vi "gnuplotVectors.vi"(0 "XYUVArray":dbl[][](array[numeric])=[[-138.0, 28.0, -5.0, -3.0], [-92.0, 28.0, -10.0, -5.5], [-46.0, 28.0, -5.0, -10.5], [0.0, 28.0, -9.0, 3.5], [46.0, 28.0, -22.0, 1.0], [92.0, 28.0, -24.5, -9.0], [138.0, 28.0, -16.0, -23.0], [-138.0, 60.0, -6.0, -2.0], [-92.0, 60.0, -7.0, -12.0], [-46.0, 60.0, -6.0, -11.0], [0.0, 60.0, -9.0, 3.0], [46.0, 60.0, -5.5, 6.0], [92.0, 60.0, -10.0, -7.5], [138.0, 60.0, -17.0, -22.0], [-138.0, 92.0, 0.5, 2.0], [-92.0, 92.0, -1.5, -15.0], [-46.0, 92.0, -1.5, -10.5], [0.0, 92.0, 1.0, -1.5], [46.0, 92.0, 1.0, 3.0], [92.0, 92.0, -2.5, -7.5], [138.0, 92.0, -5.0, -17.0], [-138.0, 124.0, 18.5, 15.0], [-92.0, 124.0, 10.5, -2.5], [-46.0, 124.0, 6.5, -2.0], [0.0, 124.0, 7.5, 5.0], [46.0, 124.0, 9.5, 12.5], [92.0, 124.0, 14.0, 8.5], [138.0, 124.0, 6.5, -4.0], [-138.0, 156.0, 13.5, 14.5], [-92.0, 156.0, 19.5, 4.0], [-46.0, 156.0, 12.5, -1.0], [0.0, 156.0, 10.5, 3.5], [46.0, 156.0, 14.0, 11.0], [92.0, 156.0, 17.5, 10.5], [138.0, 156.0, 12.0, -4.5], [-138.0, 188.0, 9.0, 16.5], [-92.0, 188.0, 10.0, 8.0], [-46.0, 188.0, 14.0, 4.0], [0.0, 188.0, 15.5, 8.0], [46.0, 188.0, 14.5, 11.0], [92.0, 188.0, 21.5, 11.0], [138.0, 188.0, 19.0, 0.5], [-138.0, 214.0, 12.5, 11.5], [-92.0, 214.0, 17.5, 6.0], [-46.0, 214.0, 17.0, 9.5], [0.0, 214.0, 14.5, 10.5], [46.0, 214.0, 19.0, 10.5], [92.0, 214.0, 20.0, 7.0], [138.0, 214.0, 16.5, 7.0]] caption="X                    Y                      U                  V", 1 "Job Directory":path) -> (2 "Saved Automatically?":bool, 3 "gnuplotScript":string, 4 "Plot data file":path)   [LabVIEW 2013]
uses:
  Results_plotter_Global.vi
panel:
  in  "OpenLogfile?":bool
  in  "Show Script Editor?":bool
  in  "Tab Control":enum32{"Titles", "OtherStuff ", "TerminalTest"}(tab)=enum."OtherStuff "
  in  "Page Title Pre Block":string
  in  "Page Title Post Block":string
  in  "Values to include in Page Title":i32[](listbox)
  out "Final Title":string
  in  "Filename Max length":i32=255
  out "File Path Control":path
  out "AuditTrail":string[](array[string])
  # "Overall Page Title"
  # "Shows the numbered line colours and point styles available- well it would, if it didn't disappear every time I update from the repository..!"
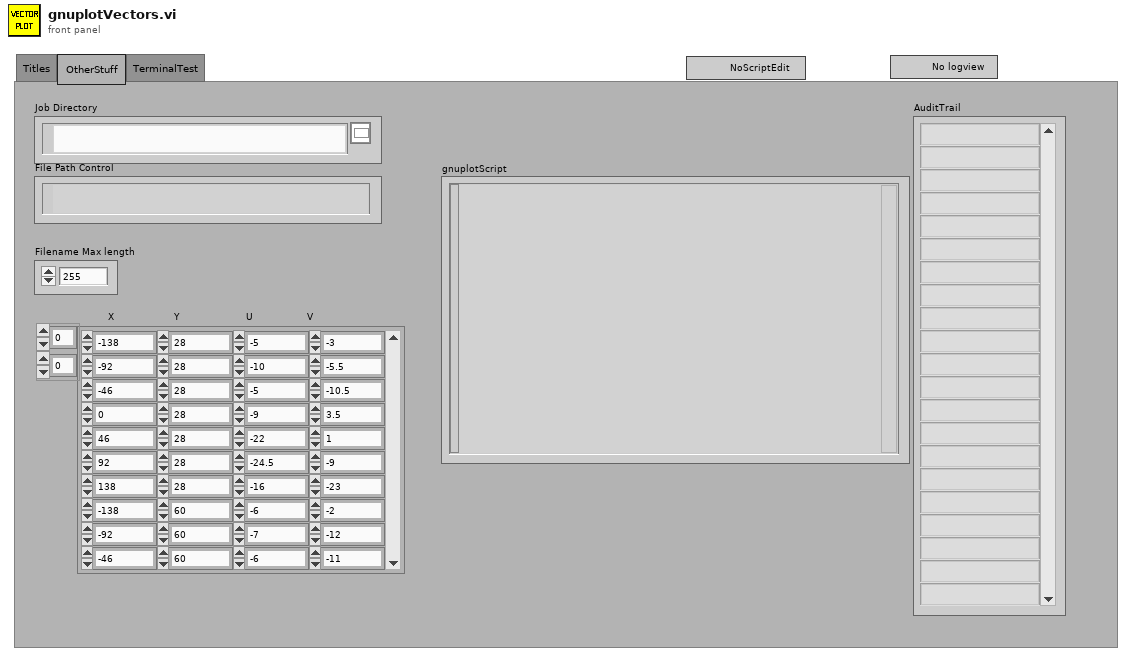
[diagram p1: front panel]
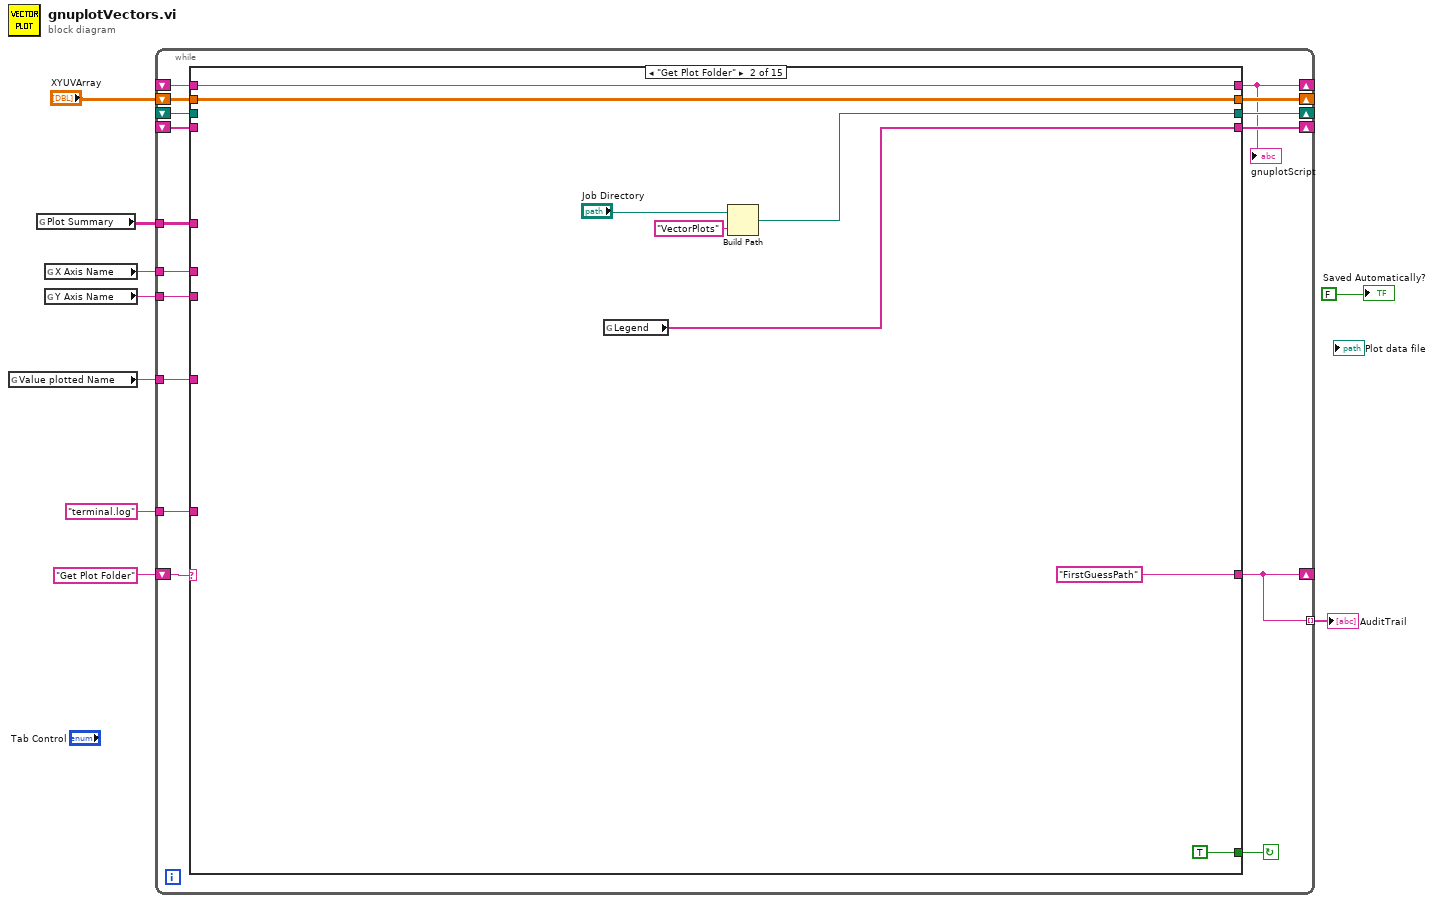
[diagram p0: block diagram]
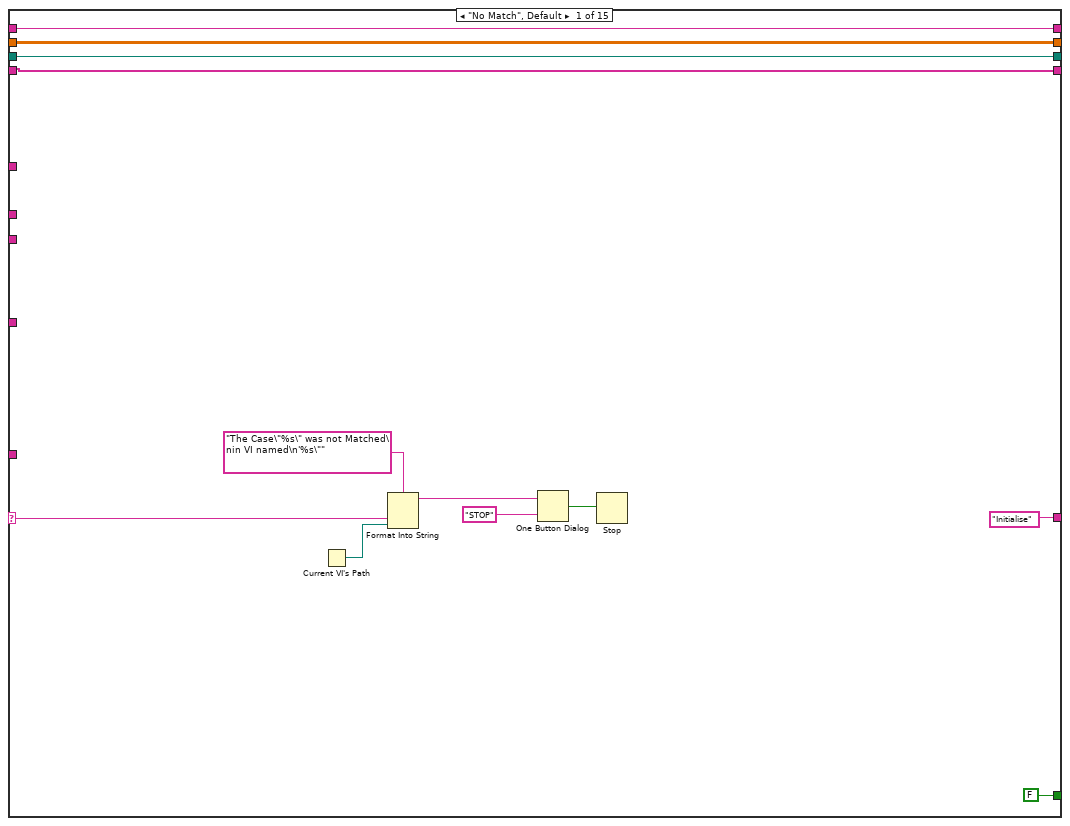
[diagram p2: hidden frame]
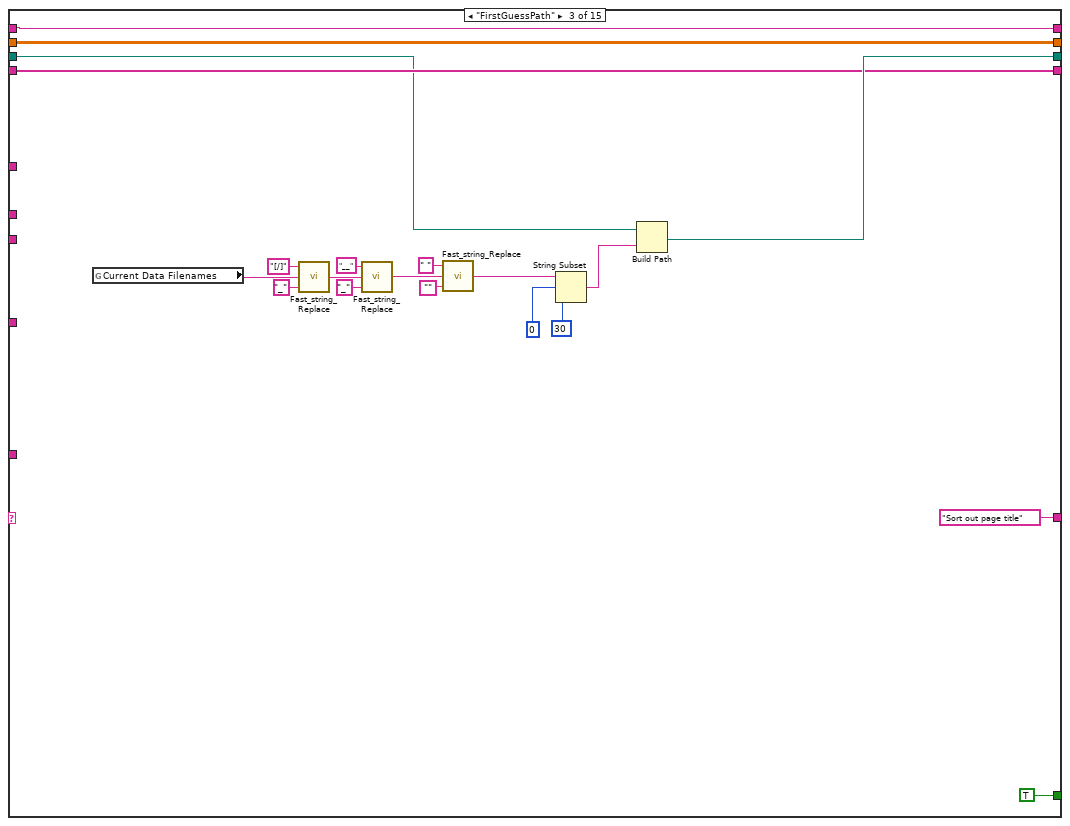
[diagram p3: hidden frame]
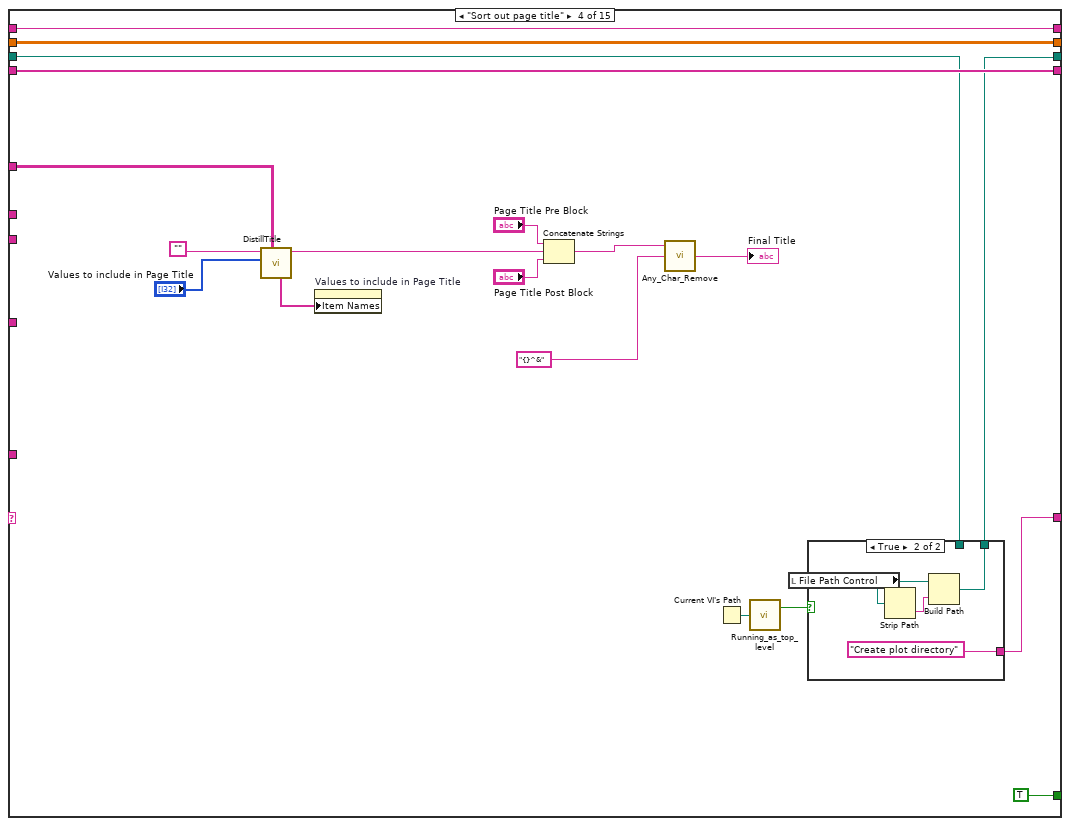
[diagram p4: hidden frame]
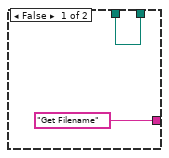
[diagram p5: hidden frame]
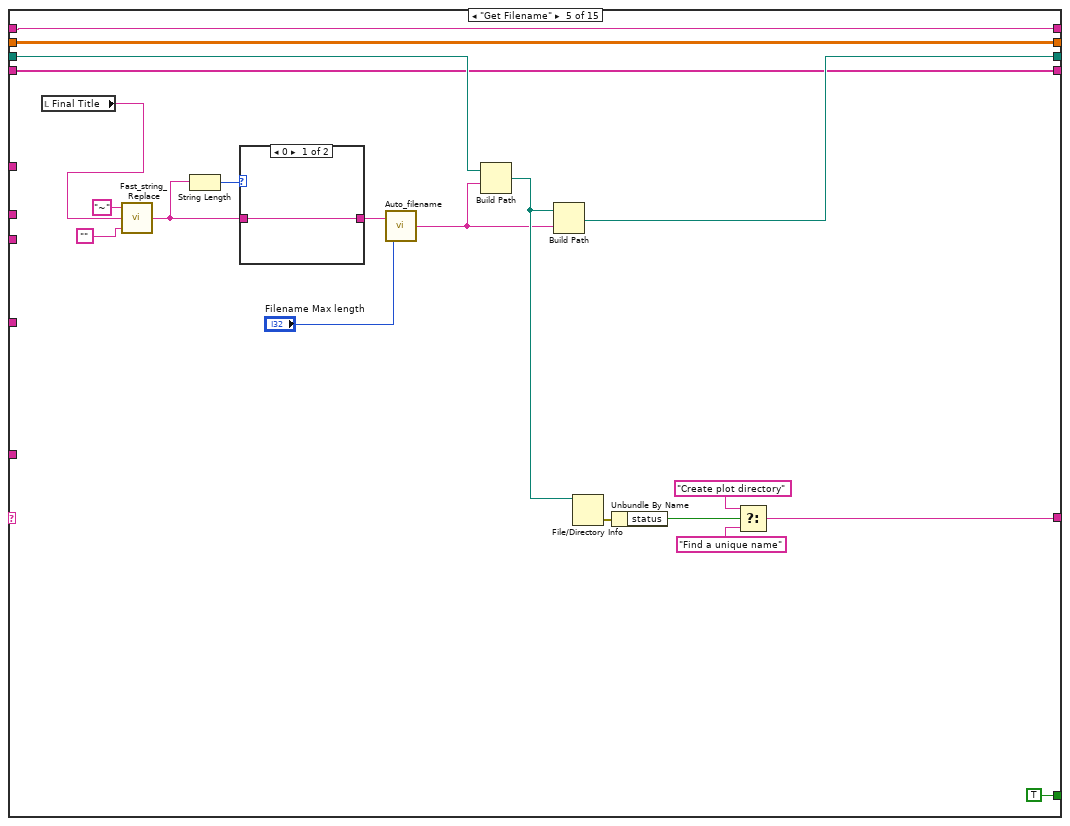
[diagram p6: hidden frame]
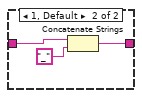
[diagram p7: hidden frame]
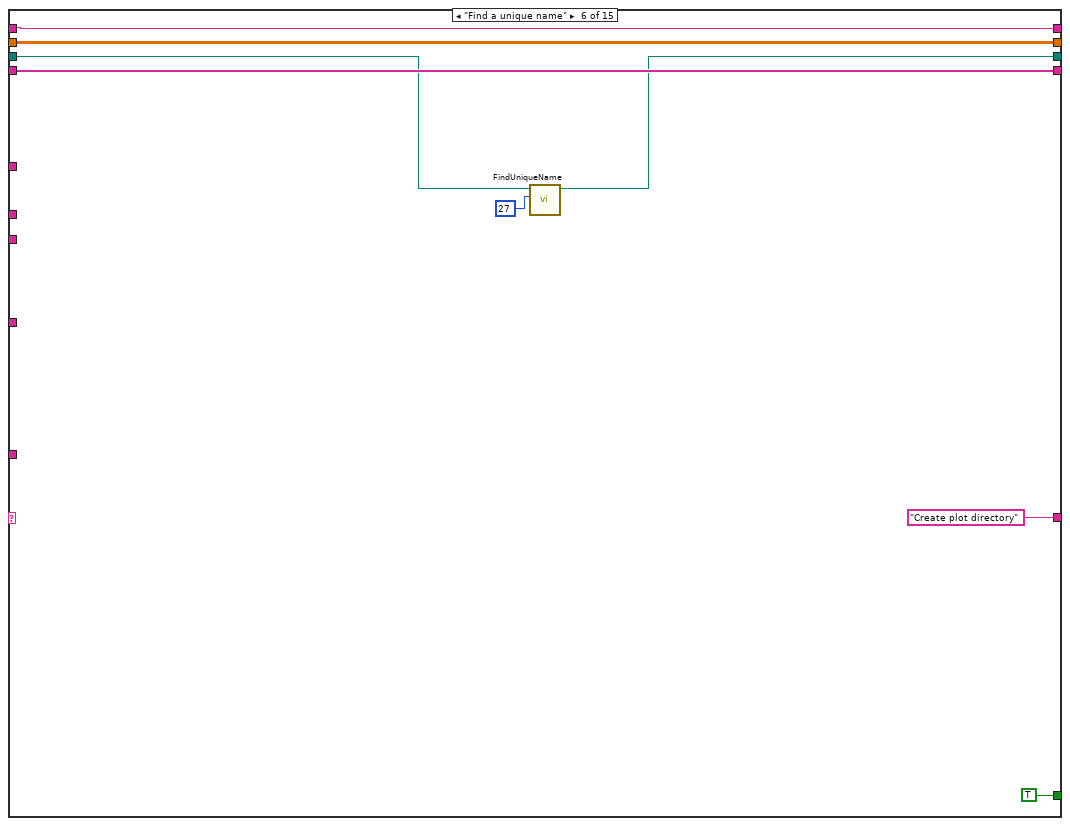
[diagram p8: hidden frame]
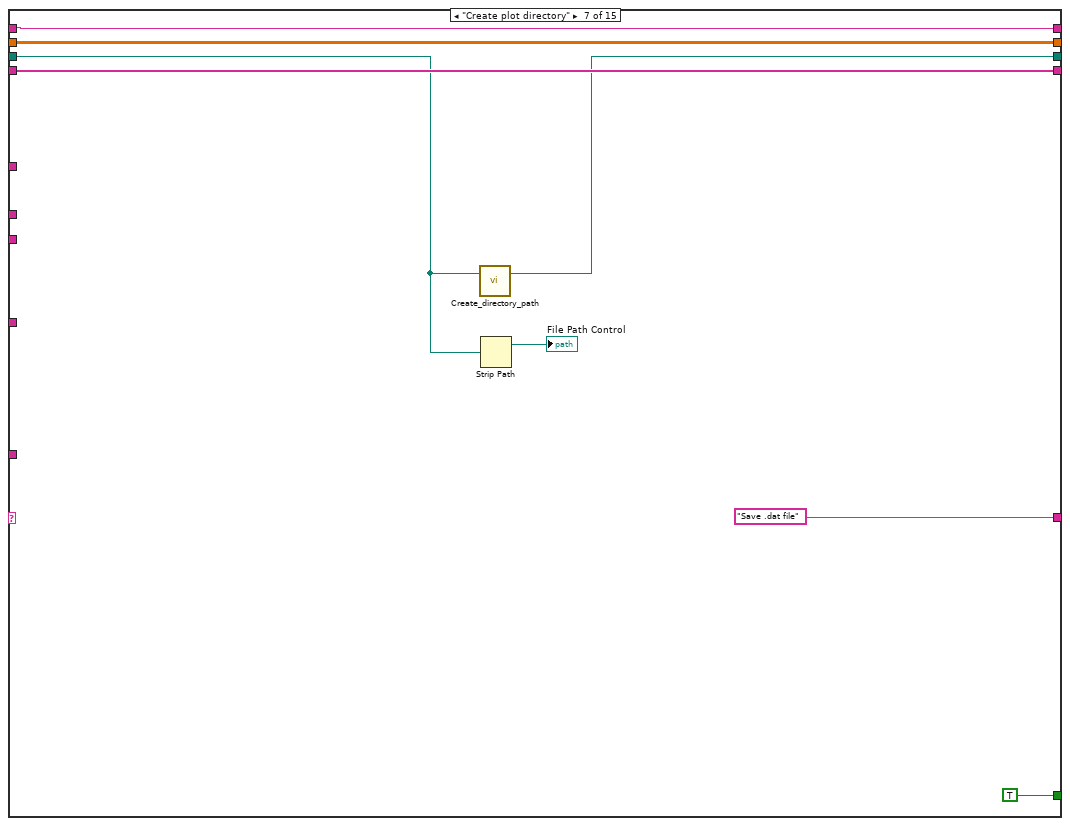
[diagram p9: hidden frame]
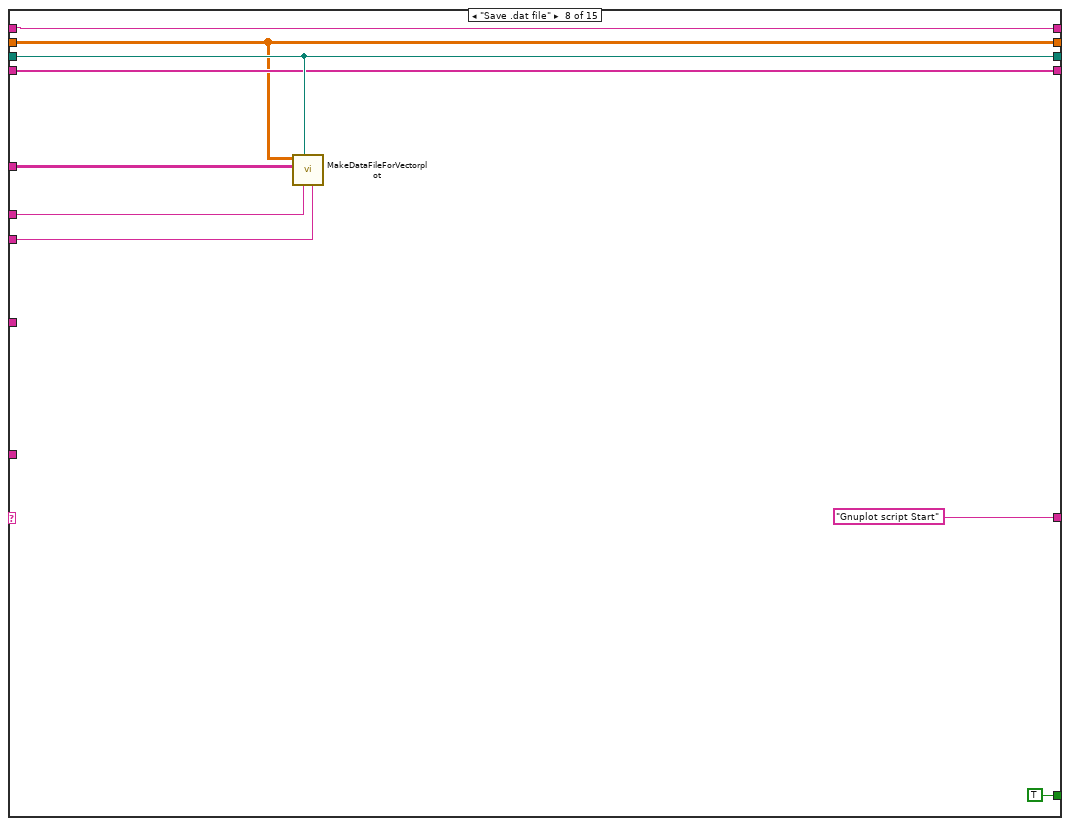
[diagram p10: hidden frame]
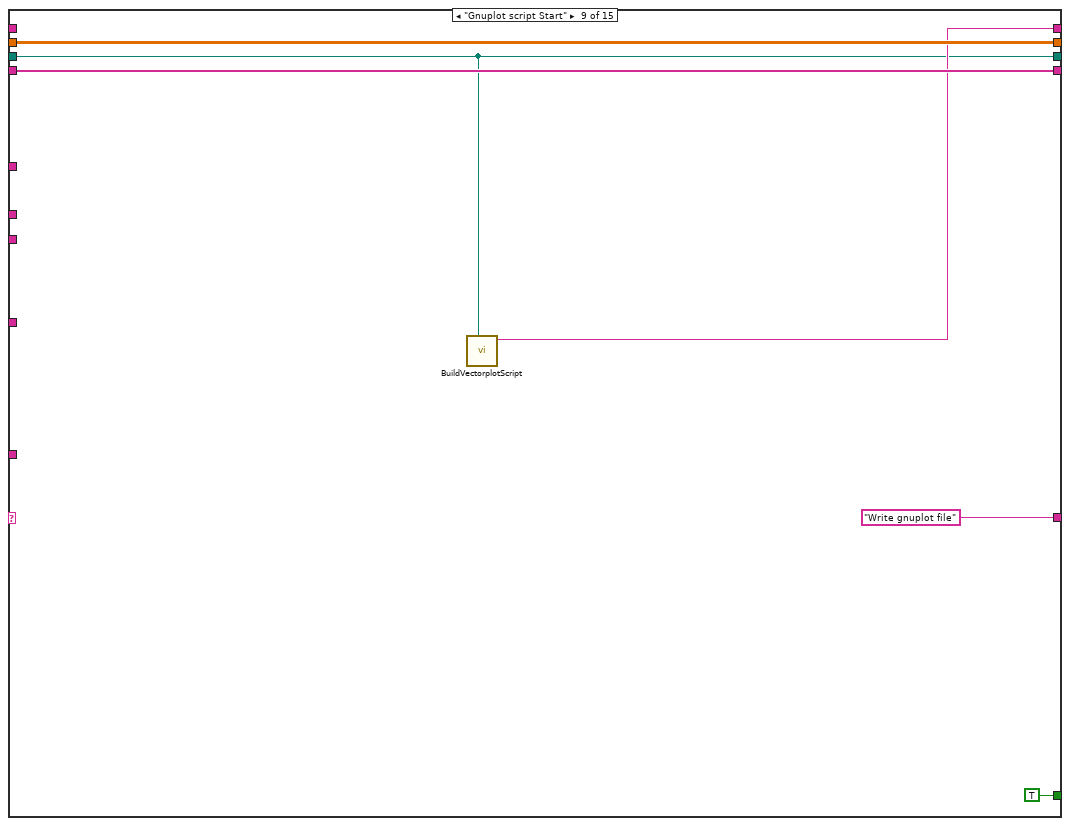
[diagram p11: hidden frame]
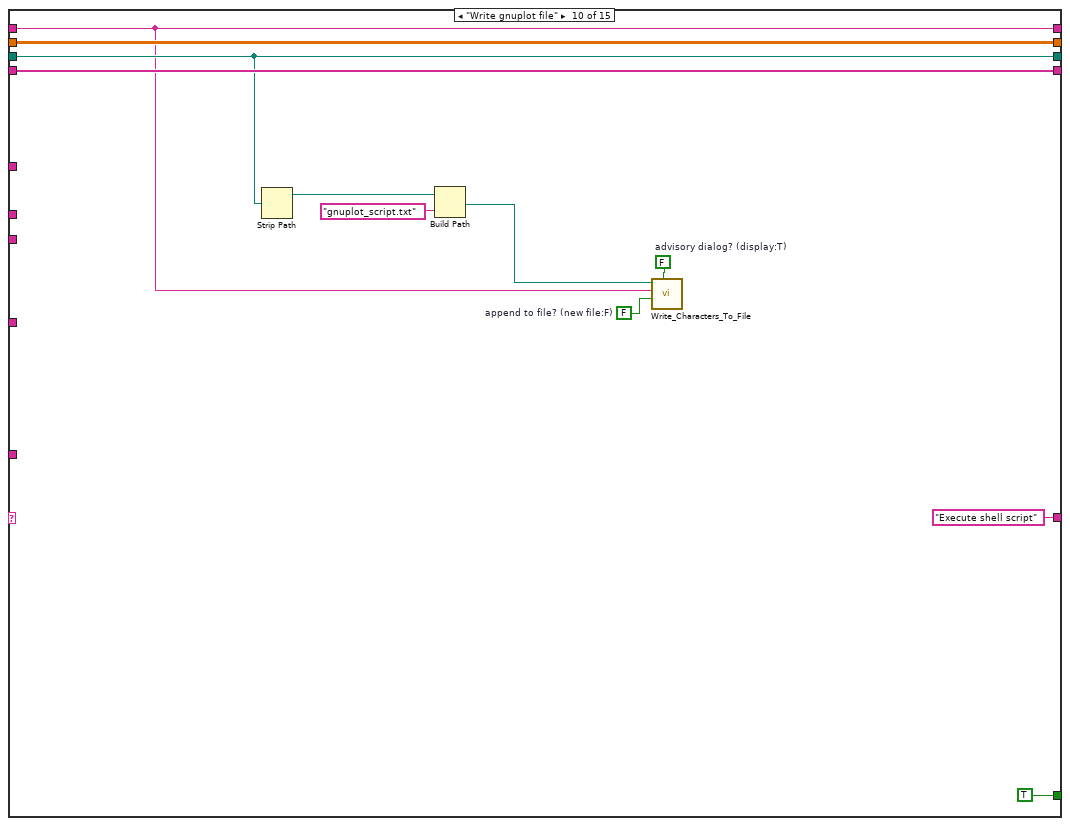
[diagram p12: hidden frame]
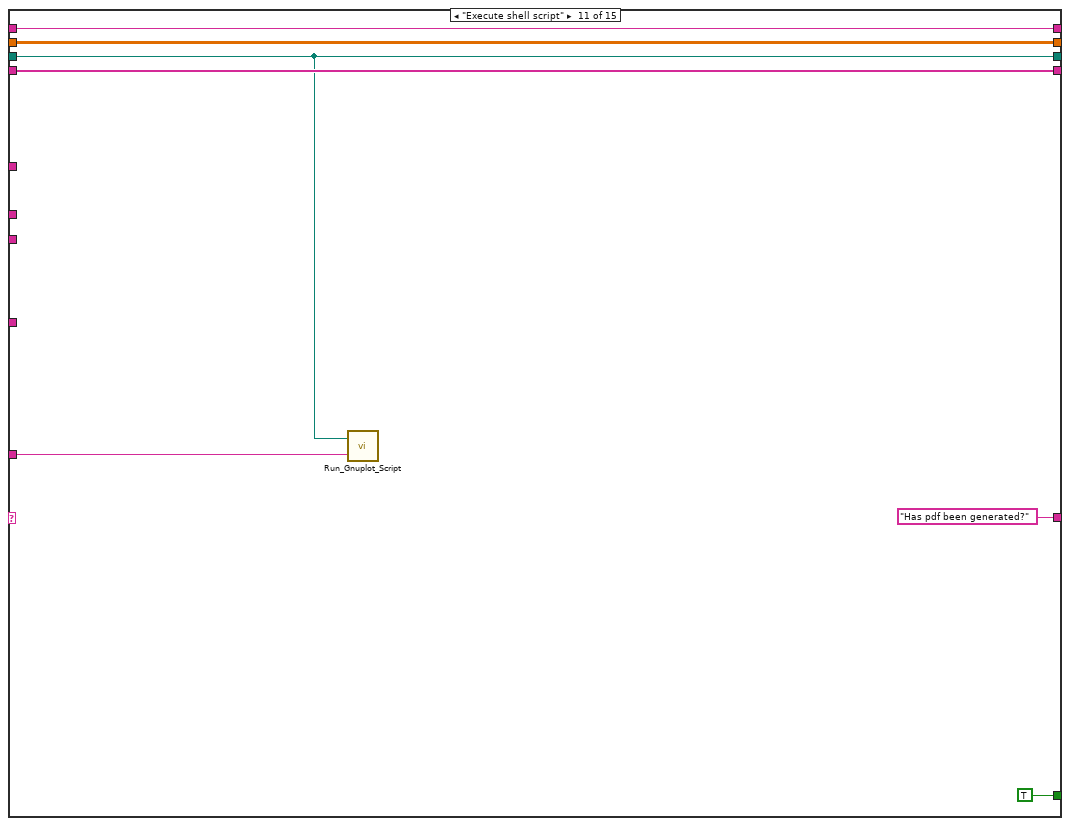
[diagram p13: hidden frame]
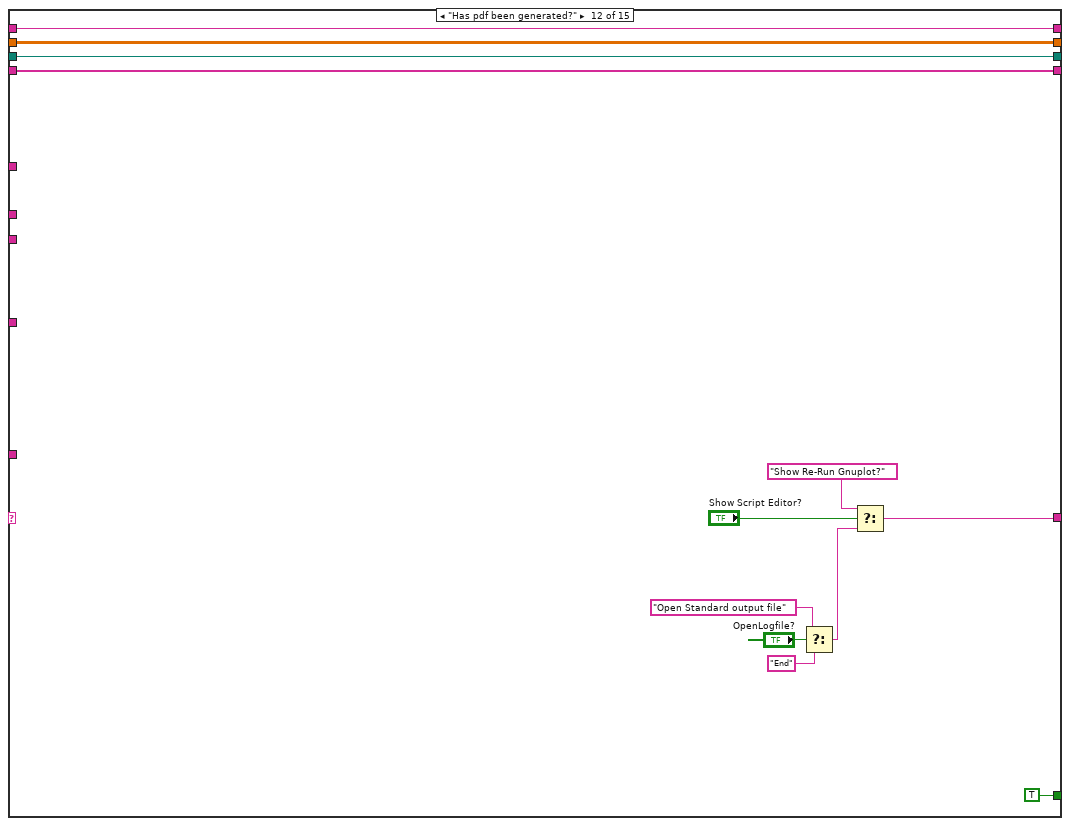
[diagram p14: hidden frame]
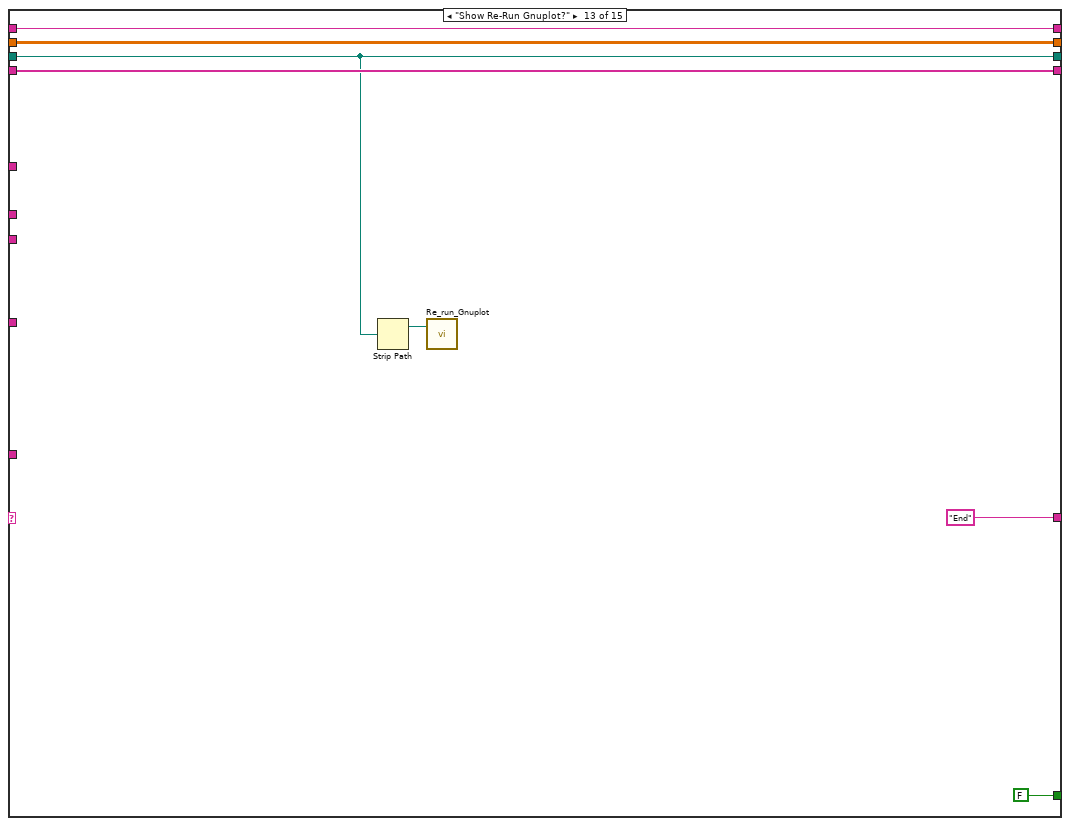
[diagram p15: hidden frame]
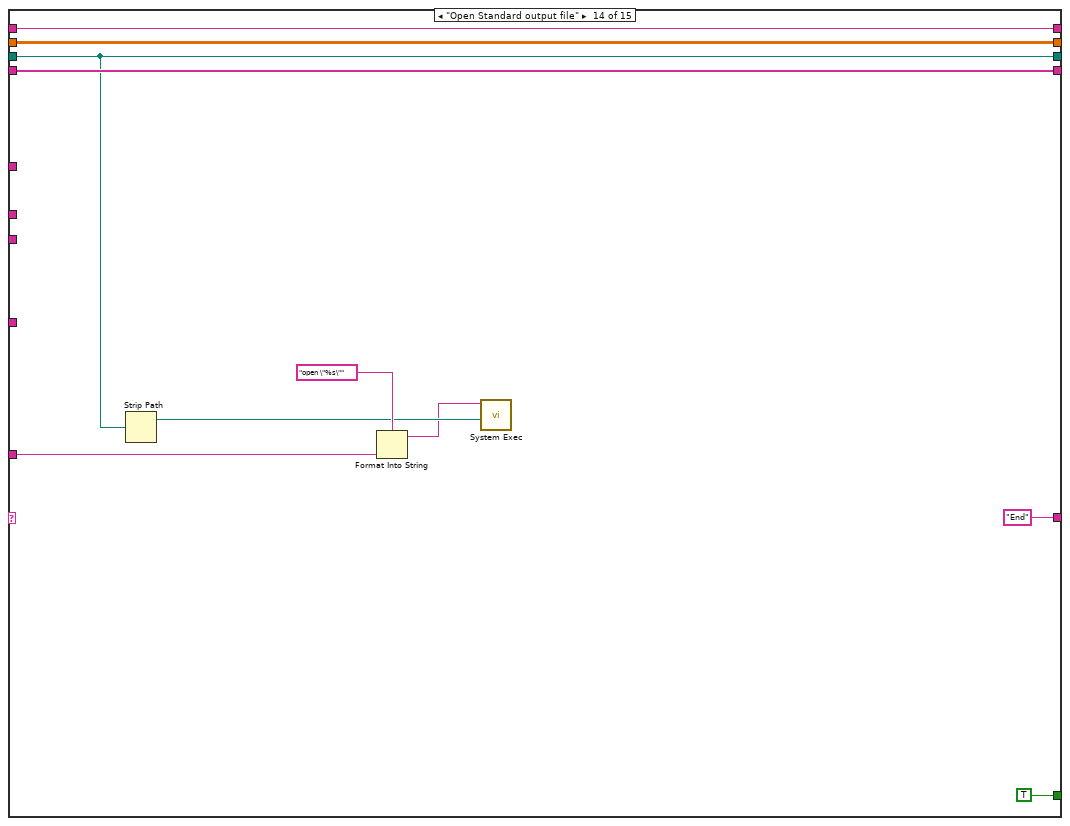
[diagram p16: hidden frame]
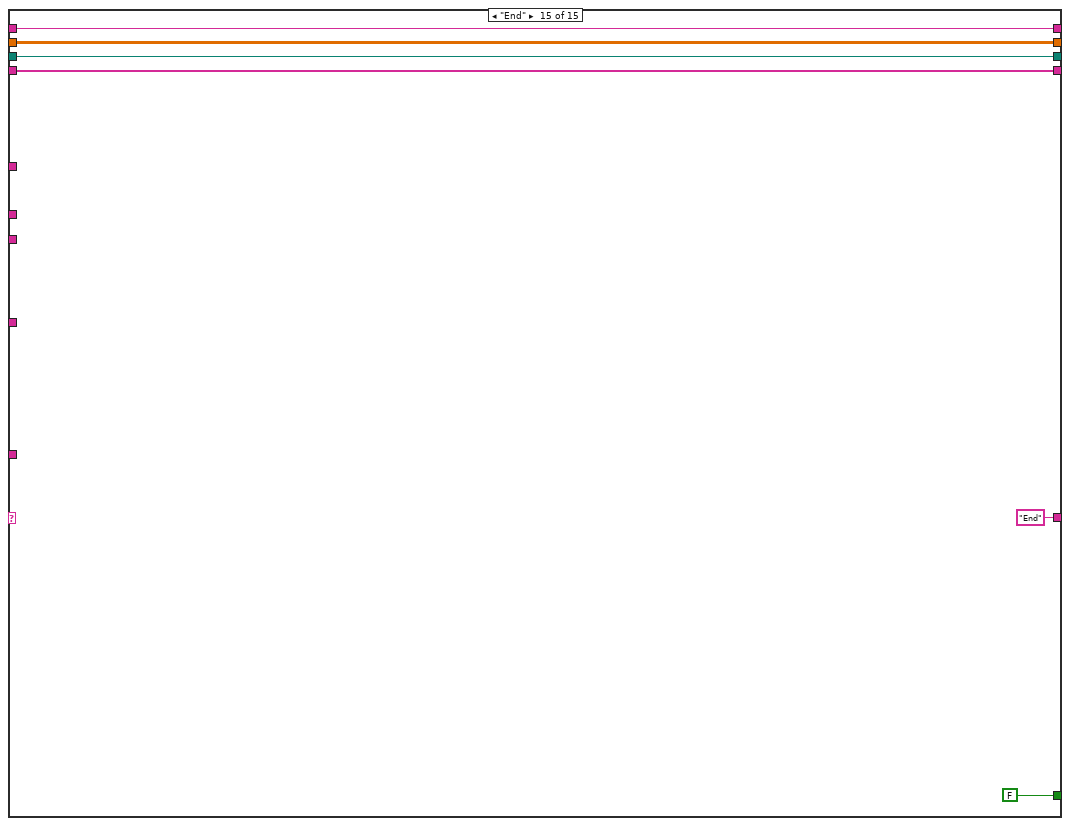
[diagram p17: hidden frame]
diagram:
  n1 = global read "Results_plotter_Global.vi" "Value plotted Name"() -> (w5:string)
  n2 = global read "Results_plotter_Global.vi" "Plot Summary"() -> (w8:string[][])
  n3 = global read "Results_plotter_Global.vi" "X Axis Name"() -> (w7:string)
  n4 = global read "Results_plotter_Global.vi" "Y Axis Name"() -> (w6:string)
  n5 = while {
    shift-left: "Get Plot Folder" -> [w24]
    shift-right: [w10] -> _
    tunnel: w8 -> [w23]
    shift-right: [w22] -> _
    shift-left: _ -> [w21]
    tunnel: w7 -> [w20]
    tunnel: w6 -> [w19]
    tunnel: w5 -> [w18]
    shift-right: [w16] -> _
    shift-left: "XYUVArray" -> [w17]
    shift-right: [w11] -> _
    shift-left: _ -> [w15]
    shift-right: [w14] -> _
    shift-left: _ -> [w13]
    tunnel: "terminal.log" -> [w12]
    tunnel: [w10] -> w2 mode=indexing
    stop <- w25 continue-if-true
    n6 = case shown="\"Get Plot Folder\"" w24 {
      selector: w24 -> [w26 _ _ _ _ _ _ _ _ _ _ _ _ _ _]
      tunnel: [FALSE TRUE TRUE ("Top Level") TRUE ("Top Level") TRUE ("Top Level") TRUE ("Top Level") TRUE TRUE ("Top Level") TRUE ("Top Level") TRUE ("Top Level") TRUE ("Top Level") TRUE ("Top Level") FALSE ("Top Level") TRUE ("Top Level") FALSE ("Top Level")] -> w25
      tunnel: ["Initialise" "FirstGuessPath" "Sort out page title" w76 w108 "Create plot directory" "Save .dat file" "Gnuplot script Start" "Write gnuplot file" ("t") "Execute shell script" ("t") "Has pdf been generated?" ("t") w168 "End" "End" ("t") "End" ("t")] -> w10
      tunnel: w23 -> [_ _ _ w71 _ _ _ w137 _ _ _ _ _ _ _]
      tunnel: [w30 w43 w65 w78 w109 w115 w127 w138 w140 w150 w158 w172 w177 w187 w198] -> w22
      tunnel: w21 -> [w30 _ w61 w77 w105 w116 w126 w138 w140 w150 w158 w172 w177 w187 w198]
      tunnel: w20 -> [_ _ _ _ _ _ _ w136 _ _ _ _ _ _ _]
      tunnel: w19 -> [_ _ _ _ _ _ _ w135 _ _ _ _ _ _ _]
      tunnel: w18 -> [_ _ _ _ _ _ _ _ _ _ _ _ _ _ _]
      tunnel: w17 -> [w29 w40 w64 w84 w107 w119 w130 w132 w145 w156 w163 w175 w182 w192 w197]
      tunnel: [w29 w40 w64 w84 w107 w119 w130 w132 w145 w156 w163 w175 w182 w192 w197] -> w16
      tunnel: w15 -> [w28 w42 w63 w82 w106 w118 w129 w139 _ w146 w161 w173 w180 w190 w196]
      tunnel: [w28 w42 w63 w82 w106 w118 w129 w139 w141 w146 w161 w173 w180 w190 w196] -> w11
      tunnel: [w27 w39 w62 w83 w104 w117 w128 w134 w144 w151 w162 w174 w181 w191 w195] -> w14
      tunnel: w13 -> [w27 _ w62 w83 w104 w117 w128 w134 w144 w151 w162 w174 w181 w191 w195]
      tunnel: w12 -> [_ _ _ _ _ _ _ _ _ _ w157 _ _ w185 _]
      frame "No Match", Default {
        n7 = Current VI's Path() -> (path=w32:path)
        n8 = Format Into String(format string="The Case\"%s\" was not Matched\nin VI named\n'%s\"" ("Format String"), w26, w32) -> (resulting string=w35:string)  [unwired: 2 in, 1 out]
        n9 = One Button Dialog(message=w35, button name ("OK")="STOP") -> (true=w33:bool)
        n10 = Stop(stop? (T)=w33) -> ()
      }
      frame "Get Plot Folder" {
        n11 = global read "Results_plotter_Global.vi" "Legend"() -> (w39:string[])
        n12 = Build Path(base path="Job Directory", name or relative path="VectorPlots") -> (appended path=w43:path)
      }
      frame "FirstGuessPath" {
        n13 = global read "Results_plotter_Global.vi" "Current Data Filenames"() -> (w50:string)
        n14 = call "Fast_string_Replace.vi"("Replace match with:"="_", "Input String"=w50, "regular expression"="[/]") -> ("Output String"=w54:string)  [unwired: 2 out]
        n15 = call "Fast_string_Replace.vi"("Replace match with:"="_", "Input String"=w54, "regular expression"="__") -> ("Output String"=w51:string)  [unwired: 2 out]
        n16 = call "Fast_string_Replace.vi"("Replace match with:"="", "Input String"=w51, "regular expression"=" ") -> ("Output String"=w49:string)  [unwired: 2 out]
        n17 = String Subset(string=w49, offset (0)=0, length (rest)=30 ("length (rest)")) -> (substring=w48:string)
        n18 = Build Path(base path=w61, name or relative path=w48) -> (appended path=w65:path)
      }
      frame "Sort out page title" {
        n19 = call "DistillTitle.vi"("Plot Summary in"=w71, "Indices to include in Page Title"="Values to include in Page Title", "String in"="") -> ("String out"=w75:string, "AvailableVariables"=w69:string[])  [unwired: 7 in]
        n20 = property on="Values to include in Page Title" class="LstBox (strict)"("Item Names"=w69) -> ()  [unwired: 2 in, 2 out]
        n21 = Concatenate Strings("Page Title Pre Block", w75, "Page Title Post Block") -> (w68:string)
        n22 = call "Any_Char_Remove.vi"("Individual Characters to Remove"="{}^&", "String in"=w68) -> ("String out"=→"Final Title":string)  [unwired: 1 in]
        n23 = Current VI's Path() -> (path=w81:path)
        n24 = call "Running_as_top_level.vi"("Vi path name"=w81) -> ("Top Level"=w79:bool)  [unwired: 1 out]
        n25 = case shown="True" w79 {
          tunnel: [w86 w89] -> w78
          tunnel: w77 -> [w86 _]
          tunnel: ["Get Filename" ("t") "Create plot directory"] -> w76
          frame False {
          }
          frame True {
            n26 = local read "File Path Control"() -> (w88:path)
            n27 = Strip Path(path=w88) -> (name=w87:string)  [unwired: 1 out]
            n28 = Build Path(base path=w88, name or relative path=w87) -> (appended path=w89:path)
          }
        }
      }
      frame "Get Filename" {
        n29 = local read "Final Title"() -> (w94:string)
        n30 = call "Fast_string_Replace.vi"("Replace match with:"="", "Input String"=w94, "regular expression"="~") -> ("Output String"=w91:string)  [unwired: 1 in, 1 out]
        n31 = String Length(string=w91) -> (length=w96:i32)
        n32 = case shown="0" w96 {
          tunnel: [w111 w112] -> w95
          tunnel: w91 -> [w111 w114]
          frame 0 {
          }
          frame 1, Default {
            n33 = Concatenate Strings(w114, "_") -> (w112:string)
          }
        }
        n34 = call "Auto_filename.vi"("Filename Max length"="Filename Max length", "Prefix"=w95) -> ("Filename"=w98:string)
        n35 = Build Path(base path=w105, name or relative path=w98) -> (appended path=w102:path)
        n36 = Build Path(base path=w102, name or relative path=w98) -> (appended path=w109:path)
        n37 = File/Directory Info(path=w102) -> (error out=w103:errorcluster)  [unwired: 1 in, 6 out]
        n38 = Unbundle By Name(w103) -> ("status"=w101:bool)
        n39 = Select(t="Create plot directory", s=w101, f="Find a unique name") -> (s? t:f=w108:string)
      }
      frame "Find a unique name" {
        n40 = call "FindUniqueName.vi"("Max Length"=27, "PathIn"=w116) -> ("UniquedPath"=w115:path)  [unwired: 9 in]
      }
      frame "Create plot directory" {
        n41 = call "Create_directory_path.vi"("Path name"=w126) -> ("Path name Out"=w127:path)  [unwired: 1 in, 1 out]
        n42 = Strip Path(path=w126) -> (stripped path=→"File Path Control":path)  [unwired: 1 out]
      }
      frame "Save .dat file" {
        n43 = call "MakeDataFileForVectorplot.vi"("Y Axis Name"=w135, "X Axis Name"=w136, "Path"=w138, "Plot Summary"=w137, "XYUVArray"=w132) -> ()  [unwired: 7 in]
      }
      frame "Gnuplot script Start" {
        n44 = call "BuildVectorplotScript.vi"("datafilePath"=w140) -> ("String out"=w141:string)  [unwired: 10 in]
      }
      frame "Write gnuplot file" {
        w153 = FALSE  # append to file? (new file:F)
        w154 = FALSE  # advisory dialog? (display:T)
        n45 = Strip Path(path=w150) -> (stripped path=w147:path)  [unwired: 1 out]
        n46 = Build Path(base path=w147, name or relative path="gnuplot_script.txt") -> (appended path=w155:path)
        n47 = call "Write_Characters_To_File.vi"("file path (dialog if empty)"=w155, "advisory dialog? (display:T)"=w154, "character string"=w146, "append to file? (new file:F)"=w153) -> ()  [unwired: 1 in, 4 out]
      }
      frame "Execute shell script" {
        n48 = call "Run_Gnuplot_Script.vi"("logfileName"=w157, "workingDirectory"=w158) -> ()
      }
      frame "Has pdf been generated?" {
        n49 = Select(t="Open Standard output file" ("f"), s="OpenLogfile?", f="End") -> (s? t:f=w164:string)
        n50 = Select(t="Show Re-Run Gnuplot?", s="Show Script Editor?", f=w164) -> (s? t:f=w168:string)
      }
      frame "Show Re-Run Gnuplot?" {
        n51 = Strip Path(path=w177) -> (stripped path=w176:path)  [unwired: 1 out]
        n52 = call "Re_run_Gnuplot.vi"("Plot folder (dialog if empty)"=w176) -> ()  [unwired: 4 out]
      }
      frame "Open Standard output file" {
        n53 = Strip Path(path=w187) -> (stripped path=w184:path)  [unwired: 1 out]
        n54 = Format Into String(format string="open \"%s\"", w185) -> (resulting string=w183:string)  [unwired: 2 in, 1 out]
        n55 = call <vilib>:"System Exec.vi"("working directory"=w184, "command line"=w183) -> ()  [unwired: 4 in, 6 out]
      }
      frame "End" {
      }
    }
    "gnuplotScript" <- w11
  }
  "AuditTrail" <- w2
  "Saved Automatically?" <- FALSE
